vi "Execute Job (Sync).vi"(8 "error in (no error)":errorcluster, 11 "Job in":refnum<class "Job.lvclass">) -> (0 "error out":errorcluster, 2 "Job Report":T1, 3 "Job out":refnum<class "Job.lvclass">)   [LabVIEW 2013, in "openCron.lvlib" / "Job.lvclass"]
uses:
  Job.lvclass
  Job Report -- cluster.ctl
  Job.lvclass/Job.ctl
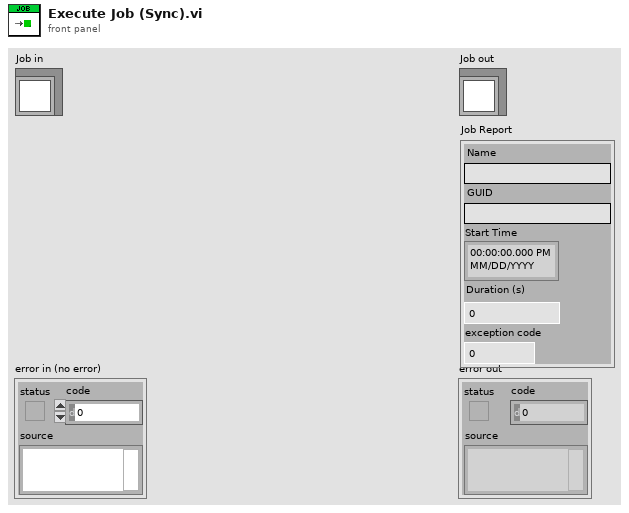
[diagram p1: front panel]
types:
  T1 = typedef "openCron.lvlib/Job.lvclass/Job Report -- cluster.ctl" = cluster{"Name":string, "GUID":string, "Start Time":timestamp, "Duration (s)":dbl, "exception code":i32}
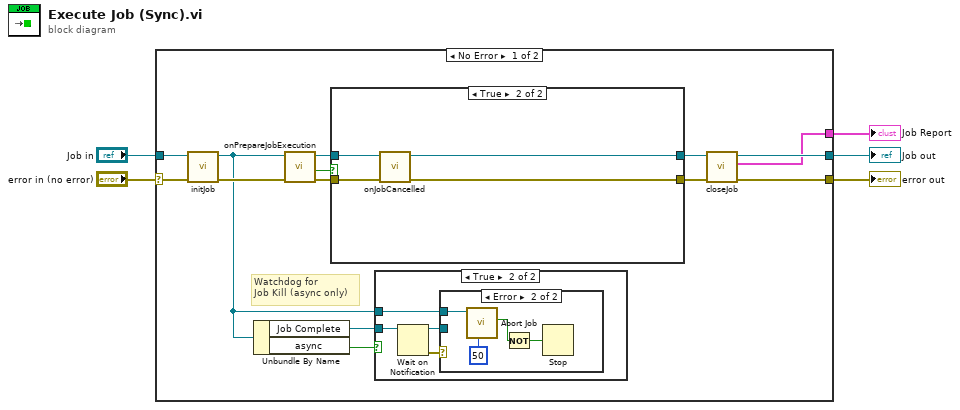
[diagram p0: block diagram]
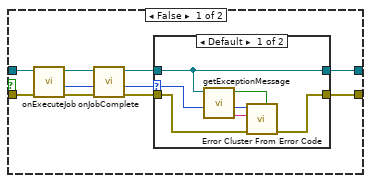
[diagram p4: hidden frame]
diagram:
  n1 = case shown="No Error" "error in (no error)" {
    selector: "error in (no error)" -> [w15 w52]
    tunnel: [w7 w51] -> w5
    tunnel: [w8 w52] -> w4
    tunnel: "Job in" -> [w16 w51]
    tunnel: [w6 _] -> w1
    frame No Error {
      # "Watchdog for\nJob Kill (async only)"
      n2 = call "initJob.vi"("error in (no error)"=w15, "Job in"=w16) -> ("error out"=w14:errorcluster, "Job out"=w9:refnum<class "Job.lvclass">)  [unwired: 8 in]
      n3 = Unbundle By Name(w9) -> ("Job Complete"=w10:refnum<notifier>, "async"=w11:bool)
      n4 = call-dynamic "onPrepareJobExecution.vi"("error in (no error)"=w14, "Job in"=w9) -> ("error out"=w18:errorcluster, "execution cancelled"=w17:bool, "Job out"=w19:refnum<class "Job.lvclass">)  [unwired: 7 in]
      n5 = case shown="True" w17 {
        tunnel: w19 -> [w28 w50]
        tunnel: w18 -> [w29 w49]
        tunnel: [w30 w47] -> w13
        tunnel: [w31 w48] -> w12
        frame False {
          n6 = call-dynamic "onExecuteJob.vi"("error in (no error)"=w29, "Job in"=w28) -> ("error out"=w36:errorcluster, "exception"=w35:i32, "Job out"=w37:refnum<class "Job.lvclass">)  [unwired: 7 in]
          n7 = call-dynamic "onJobComplete.vi"("error in (no error)"=w36, "exception"=w35, "Job in"=w37) -> ("error out"=w33:errorcluster, "unhandled exception"=w32:i32, "Job out"=w34:refnum<class "Job.lvclass">)  [unwired: 6 in]
          n8 = case shown="Default" w32 {
            selector: w32 -> [w42 _]
            tunnel: w33 -> [w44 w45]
            tunnel: w34 -> [w40 w46]
            tunnel: [w40 w46] -> w30
            tunnel: [w43 w45] -> w31
            frame Default {
              n9 = call-dynamic "getExceptionMessage.vi"("exception"=w42, "Job in"=w40) -> ("exception message"=w39:string, "exception dup"=w41:i32, "warning?"=w38:bool)  [unwired: 7 in]
              n10 = call <vilib>:"Error Cluster From Error Code.vi"("is warning? (False)"=w38, "error in (no error)"=w44, "error message (\"\")"=w39, "error code (0)"=w41) -> ("error out"=w43:errorcluster)  [unwired: 5 in]
            }
            frame 0 {
            }
          }
        }
        frame True {
          n11 = call-dynamic "onJobCancelled.vi"("error in (no error)"=w49, "Job in"=w50) -> ("error out"=w48:errorcluster, "Job out"=w47:refnum<class "Job.lvclass">)  [unwired: 8 in]
        }
      }
      n12 = case shown="True" w11 {
        tunnel: w10 -> [_ w23]
        tunnel: w9 -> [_ w20]
        frame False {
        }
        frame True {
          n13 = Wait on Notification(notifier=w23) -> (notifier out=w21:refnum<notifier>, error out=w22:errorcluster)  [unwired: 3 in, 2 out]
          n14 = case shown="Error" w22 {
            tunnel: w21 -> [_ _]
            tunnel: w20 -> [_ w27]
            frame No Error {
            }
            frame Error {
              n15 = call "Abort Job.vi"("timeout (500 ms)"=50, "Job in"=w27) -> ("Job Aborted"=w25:bool)  [unwired: 5 in, 4 out]
              n16 = Not(x=w25) -> (.not. x?=w24:bool)
              n17 = Stop(stop? (T)=w24) -> ()
            }
          }
        }
      }
      n18 = call "closeJob.vi"("error in (no error)"=w12, "Job in"=w13) -> ("error out"=w8:errorcluster, "Job Report"=w6:T1, "Job out"=w7:refnum<class "Job.lvclass">)  [unwired: 7 in]
    }
    frame Error {
    }
  }
  "error out" <- w4
  "Job out" <- w5
  "Job Report" <- w1
